vi "Config Params - Parse String Value.vi"(7 "Section":string, 8 "error in (no error)":errorcluster, 10 "Key":string, 11 "Ethernet in":refnum<class "ENET_BS1201.lvclass">) -> (0 "error out":errorcluster, 1 "Value (int)":i32, 2 "Value (dbl)":dbl, 3 "Ethernet out":refnum<class "ENET_BS1201.lvclass">, 4 "Value (bool)":bool, 5 "Value (str)":string, 6 "Found":bool)   [LabVIEW 2021, in "BS120x Driver.lvlib" / "ENET_BS1201.lvclass"]
uses:
  ENET_BS1201.lvclass
panel:
  out "ConfigurationData":string
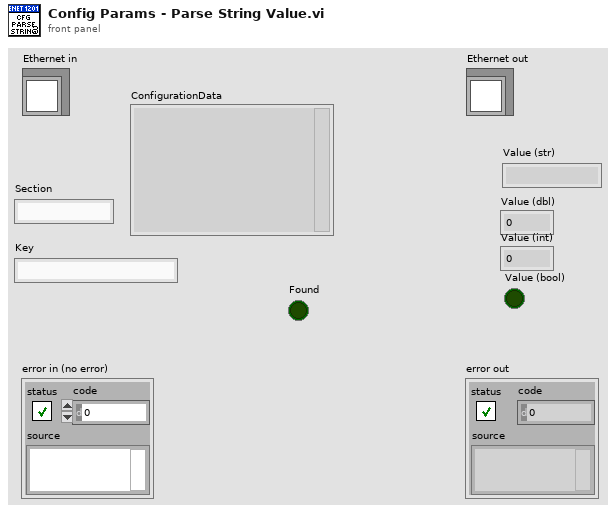
[diagram p1: front panel]
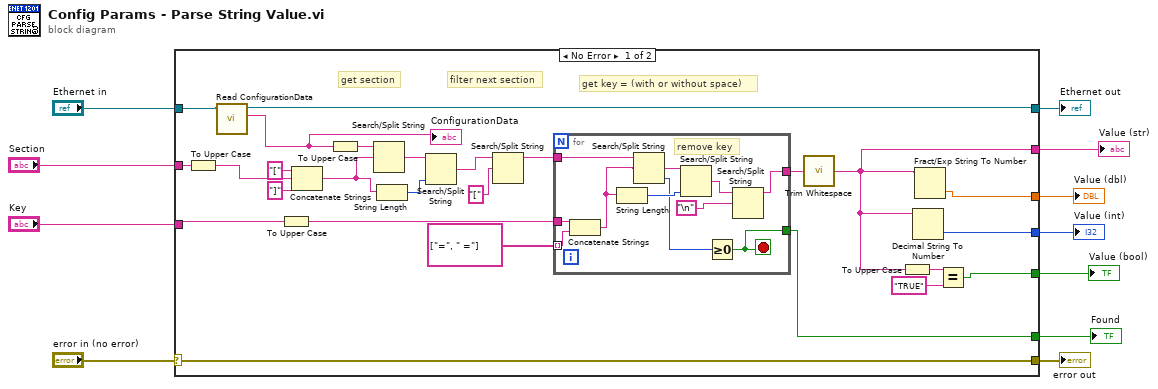
[diagram p0: block diagram]
diagram:
  n1 = case shown="No Error" "error in (no error)" {
    selector: "error in (no error)" -> [w37 w50]
    tunnel: [w37 w50] -> w10
    tunnel: [w13 w49] -> w8
    tunnel: "Ethernet in" -> [w14 w49]
    tunnel: "Section" -> [w36 _]
    tunnel: "Key" -> [w33 _]
    tunnel: [w25 _] -> w5
    tunnel: [w18 _] -> w4
    tunnel: [w24 _] -> w3
    tunnel: [w23 _] -> w2
    tunnel: [w19 _] -> w1
    frame No Error {
      # "filter next section"
      # "get key = (with or without space)"
      # "get section"
      n2 = To Upper Case(1:w36) -> (0:w16:string)
      n3 = call-dynamic "Read ConfigurationData.vi"("ENET_BS120x in"=w14) -> ("ConfigurationData"=w12:string, "ENET_BS120x out"=w13:refnum<class "ENET_BS1201.lvclass">)  [unwired: 8 in, 1 out]
      "ConfigurationData" <- w12
      n4 = To Upper Case(1:w33) -> (0:w15:string)
      n5 = Concatenate Strings("[" ("string"), w16, "]" ("string")) -> (w30:string)
      n6 = To Upper Case(1:w12) -> (0:w17:string)
      n7 = Search/Split String(string=w17, search string/char (-)=w30) -> (match + rest of string=w32:string)  [unwired: 1 in, 2 out]
      n8 = String Length(string=w30) -> (length=w31:i32)
      n9 = Search/Split String(string=w32, offset (0)=w31) -> (match + rest of string=w29:string)  [unwired: 1 in, 2 out]
      n10 = Search/Split String(string=w29, search string/char (-)="[") -> (substring before match=w27:string)  [unwired: 1 in, 2 out]
      n11 = for {
        tunnel: w27 -> [w48]
        tunnel: w15 -> [w47]
        tunnel: string[] ["=", " ="] -> [w46] mode=indexing
        tunnel: [w38] -> w22
        tunnel: [w41] -> w25
        stop <- w41 stop-if-true
        # "remove key"
        n12 = Concatenate Strings(w47, w46) -> (w43:string)
        n13 = String Length(string=w43) -> (length=w45:i32)
        n14 = Search/Split String(string=w48, search string/char (-)=w43) -> (match + rest of string=w44:string, offset of match=w42:i32)  [unwired: 1 in, 1 out]
        n15 = Search/Split String(string=w44, offset (0)=w45) -> (match + rest of string=w40:string)  [unwired: 1 in, 2 out]
        n16 = Greater Or Equal To 0?(x=w42) -> (x >= 0?=w41:bool)
        n17 = Search/Split String(string=w40, search string/char (-)="\n") -> (substring before match=w38:string)  [unwired: 1 in, 2 out]
      }
      n18 = call <vilib>:"Trim Whitespace.vi"("string"=w22) -> ("trimmed string"=w18:string)  [unwired: 1 in]
      n19 = To Upper Case(1:w18) -> (0:w21:string)
      n20 = Decimal String To Number(string=w18) -> (number=w24:i32)  [unwired: 2 in, 1 out]
      n21 = Fract/Exp String To Number(string=w18) -> (number=w23:dbl)  [unwired: 3 in, 1 out]
      n22 = Equal?(x=w21, y="TRUE") -> (x = y?=w19:bool)
    }
    frame Error {
    }
  }
  "error out" <- w10
  "Ethernet out" <- w8
  "Value (str)" <- w4
  "Value (dbl)" <- w2
  "Value (int)" <- w3
  "Value (bool)" <- w1
  "Found" <- w5
